vi "Scan stop (SubVI).vi"(8 "error in":errorcluster, 11 "VISA Refnum in":refnum<visa-resource-name>) -> (0 "error out":errorcluster, 3 "VISA Refnum out":refnum<visa-resource-name>)   [LabVIEW 2018]
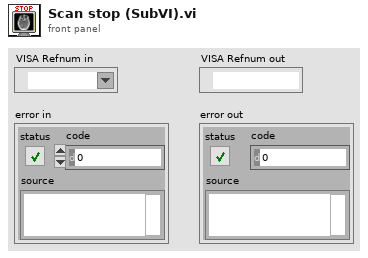
[diagram p1: front panel]
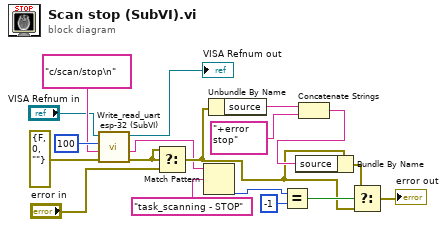
[diagram p0: block diagram]
diagram:
  n1 = call "Write_read_uart esp-32 (SubVI).vi"("error in (no error)"=errorcluster {"status"=FALSE, "code"=0, "source"=""} ("error in"), "write buffer"="c/scan/stop\n", "milliseconds to wait"=u32 100, "VISA Refnum in"="VISA Refnum in") -> ("error out 4"=w2:errorcluster, "read buffer"=w3:string, "VISA resource name out"=→"VISA Refnum out":refnum<visa-resource-name>)  [unwired: 1 out]
  n2 = Select(t=w2, s=w2, f="error in") -> (s? t:f=w4:errorcluster)
  n3 = Match Pattern(string=w3, regular expression="task_scanning - STOP") -> (offset past match=w12:i32)  [unwired: 1 in, 3 out]
  n4 = Unbundle By Name(w4) -> ("source"=w14:string)
  n5 = Equal?(x=w12, y=-1 ("offset past match")) -> (x = y?=w13:bool)
  n6 = Concatenate Strings(w14, "+error stop" ("string")) -> (w16:string)
  n7 = Bundle By Name(cluster=w4, "source"=w16) -> (w17:errorcluster)
  n8 = Select(t=w17, s=w13, f=w4) -> (s? t:f=→"error out":errorcluster)
